vi "Shooter Mode Selector.vi"(9 "Set To Manual?":bool, 10 "Set To Safe?":bool, 11 "Set To Auto?":bool) -> (3 "Mode":T1)   [LabVIEW 2015]
uses:
  Common Code/Shoot Modes Enum.ctl
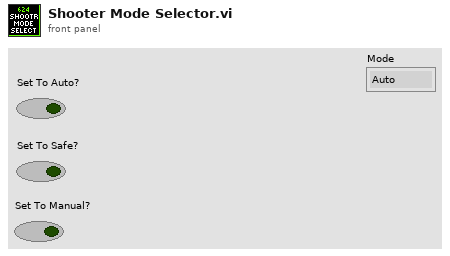
[diagram p1: front panel]
types:
  T1 = typedef "Shoot Modes Enum.ctl" = enum16{"Auto"}
  T2 = enum16{"0", "1", "2", "3", "4", "5", "6", "7", "8", "9", "A", "B", "C", "D", "E", "F", "G", "H", "I", "J", "K", "L", "M", "N", "O", "P", "Q", "R", "S", "T", "U", "V", "W", "X", "Y", "Z", "F1", "F2", "F3", "F4", "F5", "F6", "F7", "F8", "F9", "F10", "F11", "F12", "F13", "F14", "F15", "ADD", "BACK", "BACKSLASH", "CAPITAL", "COMMA", "DECIMAL", "DELETE", "DIVIDE", "DOWN", "END", "EQUALS", "ESCAPE", "GRAVE (`)", "HOME", "INSERT", "LBRACKET", "LCONTROL", "LEFT", "L ALT", "LSHIFT", "LWIN", "MINUS", "MULTIPLY", "NEXT", "NUMLOCK", "NUMPAD_0", "NUMPAD_1", "NUMPAD_2", "NUMPAD_3", "NUMPAD_4", "NUMPAD_5", "NUMPAD_6", "NUMPAD_7", "NUMPAD_8", "NUMPAD_9", "PAUSE", "PERIOD", "PRIOR (PG UP)", "RBRACKET", "RCONTROL", "RETURN", "RIGHT", "R ALT", "RSHIFT", "RWIN", "SCROLL", "SEMICOLON", "SLASH", "SPACE", "SUBTRACT", "TAB", "UP", "ENTER (num pad)", "' (quote)"}
  T3 = typedef "Shoot Modes Enum.ctl" = enum16{"Manual", "Safe", "Auto"}
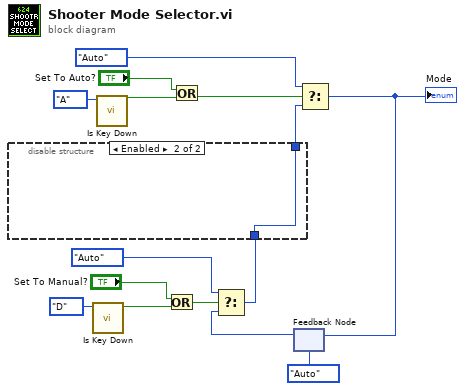
[diagram p0: block diagram]
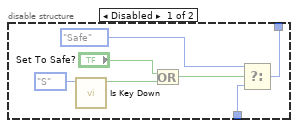
[diagram p2: hidden frame]
diagram:
  n1 = call "Is Key Down.vi"("Key"=T2."D") -> ("Key Down?"=w9:bool)  [unwired: 10 in]
  n2 = call "Is Key Down.vi"("Key"=T2."A") -> ("Key Down?"=w14:bool)  [unwired: 10 in]
  n3 = Or(x="Set To Manual?", y=w9) -> (x .or. y?=w8:bool)
  n4 = Or(x="Set To Auto?", y=w14) -> (x .or. y?=w12:bool)
  n5 = feedback #1(Shoot_Modes_Enum."Auto" ("Mode")) -> (w2:T1)
  n6 = Select(t=enum16{"Auto"}."Auto" ("Mode"), s=w8, f=w2) -> (s? t:f=w4:T1)
  n7 = disable-structure shown="Enabled" {
    disable-tunnel: [w17 w23] -> w5
    disable-tunnel: w4 -> [w16 w23]
    frame Disabled {
      n8 = call "Is Key Down.vi"("Key"=T2."S") -> ("Key Down?"=w20:bool)  [unwired: 10 in]
      n9 = Or(x="Set To Safe?", y=w20) -> (x .or. y?=w19:bool)
      n10 = Select(t=Shoot_Modes_Enum."Safe" ("Mode"), s=w19, f=w16) -> (s? t:f=w17:u16)
    }
    frame Enabled {
    }
  }
  n11 = Select(t=enum16{"Auto"}."Auto" ("Mode"), s=w12, f=w5) -> (s? t:f=w3:T1)
  "Mode" <- w3
  n12 = feedback-in #1(w3) -> ()
